vi "Stage2.vi"(0 "Start":bool, 1 "Stop":bool, 2 "Reset":bool, 3 "C":bool[][](array[boolean]), 4 "Stage table":u32[][](array[numeric])=[[0, 2, 2, 2, 2], [0, 3, 3, 3, 3], [0, 4, 4, 4, 4], [0, 0, 0, 0, 0]], 6 "Step":bool, 7 "End step":u32=4, 9 "Descriptions":string[](array[string])) -> (13 "Description":string, 14 "Start":bool, 15 "Stop":bool, 16 "End":bool, 17 "t":u32, 18 "N curr":u32)   [LabVIEW 2019]
uses:
  Logik/Logik.lvlib
  Trigers/Triggers.lvlib
  Timer Delay/Timers.lvlib
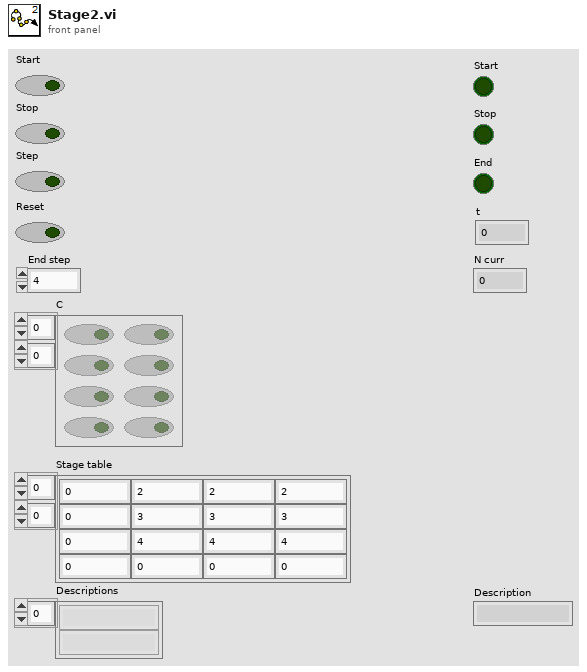
[diagram p1: front panel]
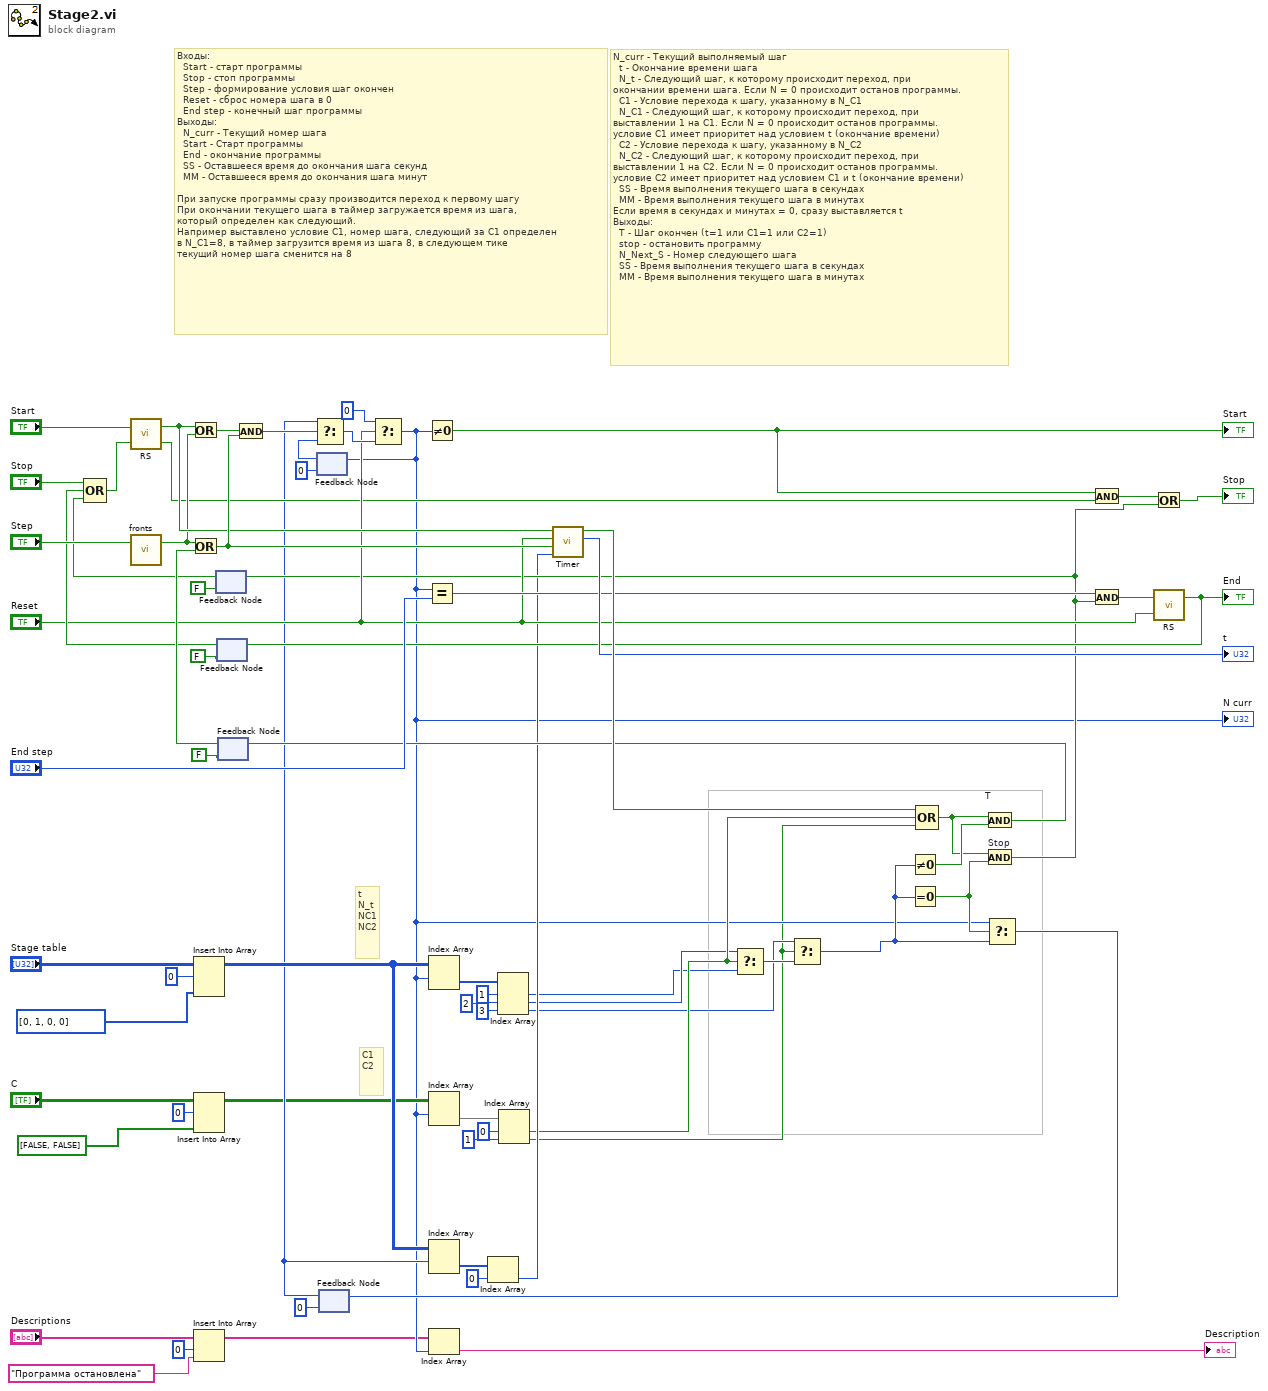
[diagram p0: block diagram]
diagram:
  # "C1\nC2"
  # "t\nN_t\nNC1\nNC2"
  # "N_curr - Текущий выполняемый шаг\n  t - Окончание времени шага\n  N_t - Следующий шаг, к которому происходит переход, при\nокончании времени шага. Если N = 0 происходит останов программы.\n  C1 - Условие перехода к шагу, указанному в N_C1\n  N_C1 - Следующий шаг, к которому происходит переход, при\nвыставлении 1 на С1. Если N = 0 происходит останов программы.\nусловие С1 имеет приоритет над условием t (окончание времени)\n  C2 - Условие перехода к шагу, указанному в N_C2\n  N_C2 - Следующий шаг, к которому происходит переход, при\nвыставлении 1 на С2. Если N = 0 происходит останов программы.\nусловие С2 имеет приоритет над условием С1 и t (окончание времени)\n  SS - Время выполнения текущего шага в секундах\n  MM - Время выполнения текущего шага в минутах\nЕсли время в секундах и минутах = 0, сразу выставляется t\nВыходы:\n  T - Шаг окончен (t=1 или C1=1 или С2=1)\n  stop - остановить программу\n  N_Next_S - Номер следующего шага\n  SS - Время выполнения текущего шага в секундах\n  MM - Время выполнения текущего шага в минутах"
  # "Входы:\n  Start - старт программы\n  Stop - стоп программы\n  Step - формирование условия шаг окончен\n  Reset - сброс номера шага в 0\n  End step - конечный шаг программы\nВыходы:\n  N_curr - Текущий номер шага\n  Start - Старт программы\n  End - окончание программы\n  SS - Оставшееся время до окончания шага секунд\n  MM - Оставшееся время до окончания шага минут\n\nПри запуске программы сразу производится переход к первому шагу\nПри окончании текущего шага в таймер загружается время из шага,\nкоторый определен как следующий.\nНапример выставлено условие C1, номер шага, следующий за С1 определен\nв N_C1=8, в таймер загрузится время из шага 8, в следующем тике \nтекущий номер шага сменится на 8"
  n1 = call "fronts.vi"("in"="Step") -> ("raise"=w58:bool)  [unwired: 1 in, 1 out]
  n2 = Insert Into Array(array="Stage table", index (row)=0 ("index"), new element=u32[] [0, 1, 0, 0]) -> (w43:u32[][])  [unwired: 1 in]
  n3 = Insert Into Array(array="C", index (row)=0, new element=bool[] [FALSE, FALSE]) -> (w18:bool[][])  [unwired: 1 in]
  n4 = Insert Into Array(array="Descriptions", index=0, new element="Программа остановлена" ("new element/subarray")) -> (w8:string[])
  n5 = feedback #1(FALSE ("Q")) -> (w48:bool)
  n6 = feedback #2(FALSE ("Q")) -> (w47:bool)
  n7 = Compound Arithmetic op=OR("Stop", w47, w48) -> (w67:bool)
  n8 = call "RS.vi"("R"=w67, "S"="Start") -> ("~Q"=w32:bool, "Q"=w60:bool)
  n9 = Or(x=w60, y=w58) -> (x .or. y?=w69:bool)
  n10 = feedback #3(FALSE ("Q")) -> (w50:bool)
  n11 = Or(x=w58, y=w50) -> (x .or. y?=w61:bool)
  n12 = And(x=w69, y=w61) -> (x .and. y?=w68:bool)
  n13 = feedback #4(u32 0) -> (w40:u32)
  n14 = feedback #5(u32 0) -> (w27:u32)
  n15 = Select(t=w27, s=w68, f=w40) -> (s? t:f=w42:u32)
  n16 = Select(t=u32 0, s="Reset", f=w42) -> (s? t:f=w13:u32)
  "N curr" <- w13
  n17 = feedback-in #4(w13) -> ()
  n18 = Not Equal To 0?(x=w13) -> (x != 0?=w38:bool)
  "Start" <- w38
  n19 = Equal?(x=w13, y="End step") -> (x = y?=w35:bool)
  n20 = Index Array(array=w43, index (row)=w13) -> (element=w22:u32[])  [unwired: 1 in]
  n21 = Index Array(array=w18, index (row)=w13) -> (element=w17:bool[])  [unwired: 1 in]
  n22 = Index Array(array=w43, index (row)=w27) -> (element=w26:u32[])  [unwired: 1 in]
  n23 = Index Array(array=w8, index=w13) -> (element=→"Description":string)
  n24 = Index Array(array=w26, index=0) -> (element=w25:u32)
  n25 = Index Array(array=w22, index #1=1 ("index"), index #2=2 ("index"), index #3=3 ("index")) -> (element #1=w3:u32, element #2=w4:u32, element #3=w7:u32)
  n26 = Index Array(array=w17, index #1=0 ("index"), index #2=1 ("index")) -> (element #1=w15:bool, element #2=w1:bool)
  n27 = call "Timer.vi"("ms"=w25, "Load (F)"=w61, "Reset (F)"="Reset", "Start (T)"=w60) -> ("t ms"=→"t":u32, "End"=w53:bool)  [unwired: 5 in]
  n28 = Select(t=w4, s=w15, f=w3) -> (s? t:f=w57:u32)
  n29 = Select(t=w7, s=w1, f=w57) -> (s? t:f=w14:u32)
  n30 = Not Equal To 0?(x=w14) -> (x != 0?=w56:bool)
  n31 = Equal To 0?(x=w14) -> (x = 0?=w54:bool)
  n32 = Compound Arithmetic op=OR(w53, w15, w1) -> (w55:bool)
  n33 = And "T"(x=w55, y=w56) -> (x .and. y?=w51:bool)
  n34 = feedback-in #3(w51) -> ()
  n35 = And "Stop"(x=w55, y=w54) -> (x .and. y?=w31:bool)
  n36 = feedback-in #1(w31) -> ()
  n37 = Select(t=w13, s=w54, f=w14) -> (s? t:f=w44:u32)
  n38 = feedback-in #5(w44) -> ()
  n39 = And(x=w38, y=w32) -> (x .and. y?=w34:bool)
  n40 = And(x=w35, y=w31) -> (x .and. y?=w63:bool)
  n41 = Or(x=w34, y=w31) -> (x .or. y?=→"Stop":bool)
  n42 = call "RS.vi"("R"="Reset", "S"=w63) -> ("Q"=w36:bool)  [unwired: 1 out]
  "End" <- w36
  n43 = feedback-in #2(w36) -> ()
